vi "COMMAND_ChangeVelocity.vi"(8 "error in (no error)":errorcluster, 10 "velocity":dbl[unit], 11 "StageDL090602SutterMP285 in":refnum<class "StageMMS2015ASI.lvclass">) -> (0 "error out":errorcluster, 3 "StageDL090602SutterMP285 out":refnum<class "StageMMS2015ASI.lvclass">)   [LabVIEW 2010, in "StageMMS2015ASI.lvclass"]
uses:
  StageMMS2015ASI.lvclass
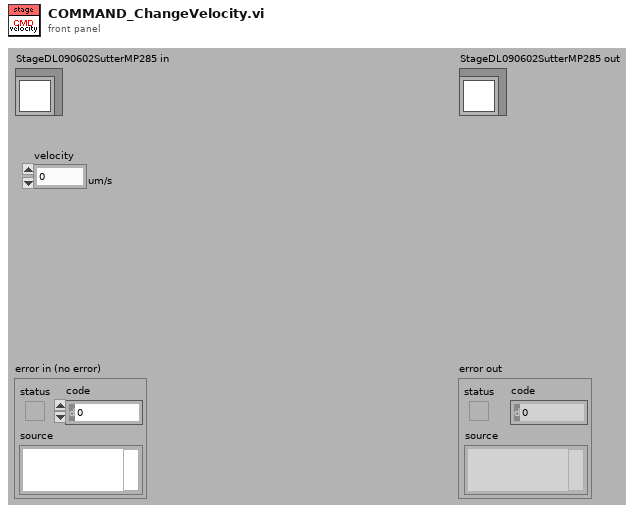
[diagram p1: front panel]
types:
  T1 = typedef "StageMMS2015ASI.lvclass/status_cluster.ctl" = cluster{"STEP_DIV":i32, "STEP_MUL":i32, "XSPEED":i32, "VERSION":i32}
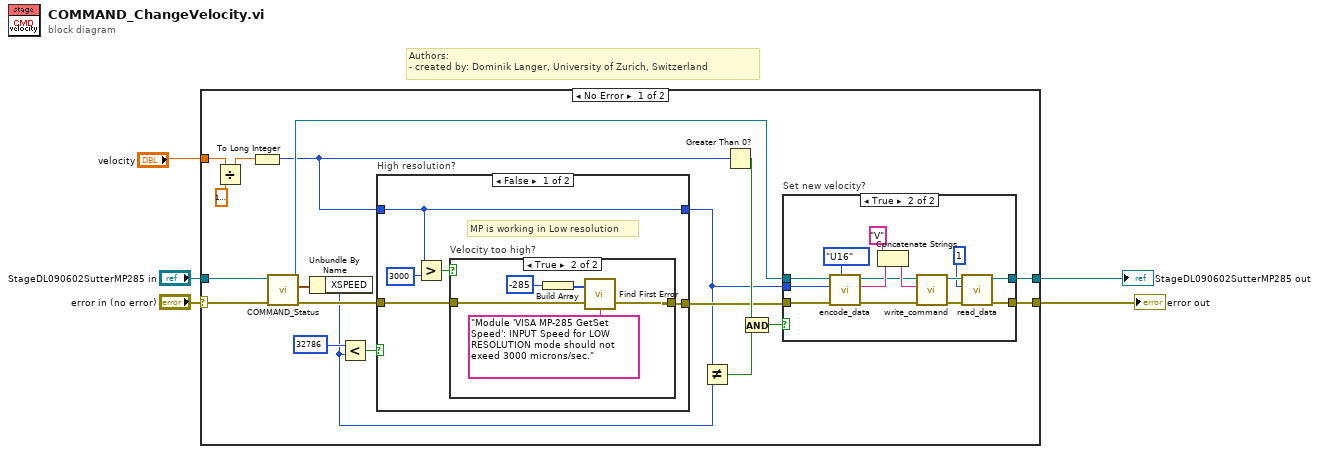
[diagram p0: block diagram]
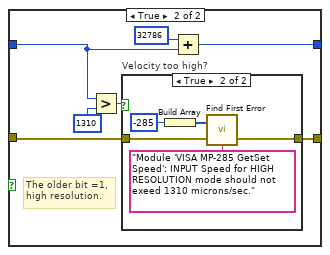
[diagram p4: hidden frame]
diagram:
  # "Authors: \n- created by: Dominik Langer, University of Zurich, Switzerland"
  n1 = case shown="No Error" "error in (no error)" {
    selector: "error in (no error)" -> [w24 w66]
    tunnel: [w22 w66] -> w4
    tunnel: [w21 w65] -> w2
    tunnel: "StageDL090602SutterMP285 in" -> [w23 w65]
    tunnel: "velocity" -> [w9 _]
    frame No Error {
      n2 = Divide(x=w9, y=dbl[unit] 1e-06) -> (x/y=w8:dbl)
      n3 = To Long Integer(number=w8) -> (32bit integer=w7:i32)
      n4 = call-dynamic "COMMAND_Status.vi"("error in (no error)"=w24, "StageDL090602SutterMP285 in"=w23) -> ("error out"=w14:errorcluster, "status"=w20:T1, "StageDL090602SutterMP285 out"=w11:refnum<class "StageMMS2015ASI.lvclass">)  [unwired: 7 in]
      n5 = Unbundle By Name(w20) -> ("XSPEED"=w12:i32)
      n6 = Less?(x=32786, y=w12) -> (x < y?=w19:bool)
      n7 = case "High resolution?" shown="False" w19 {
        tunnel: [w41 w53] -> w6
        tunnel: w7 -> [w41 w52]
        tunnel: w14 -> [w43 w55]
        tunnel: [w42 w54] -> w13
        frame False {
          # "MP is working in Low resolution"
          n8 = Greater?(x=w41, y=3000) -> (0:w44:bool)
          n9 = case "Velocity too high?" shown="True" w44 {
            tunnel: w43 -> [w46 w51]
            tunnel: [w46 w50] -> w42
            frame False {
              # "An INPUT is\nin range."
            }
            frame True {
              n10 = Build Array(-285) -> (w49:i32[])
              n11 = call <vilib>:"Find First Error.vi"("error in (no error)"=w51, "source messages"="Module 'VISA MP-285 GetSet Speed': INPUT Speed for LOW RESOLUTION mode should not exeed 3000 microns/sec.", "error codes"=w49) -> ("error out"=w50:errorcluster)  [unwired: 1 in, 1 out]
            }
          }
        }
        frame True {
          # "The older bit =1, \nhigh resolution."
          n12 = Greater?(x=w52, y=1310) -> (0:w57:bool)
          n13 = case "Velocity too high?" shown="True" w57 {
            tunnel: w55 -> [w59 w63]
            tunnel: [w59 w64] -> w54
            frame False {
              # "Input correct, \nWe can write."
            }
            frame True {
              n14 = Build Array(-285) -> (w61:i32[])
              n15 = call <vilib>:"Find First Error.vi"("error in (no error)"=w63, "source messages"="Module 'VISA MP-285 GetSet Speed': INPUT Speed for HIGH RESOLUTION mode should not exeed 1310 microns/sec.", "error codes"=w61) -> ("error out"=w64:errorcluster)  [unwired: 1 in, 1 out]
            }
          }
          n16 = Add(x=32786, y=w52) -> (x+y=w53:i32)
        }
      }
      n17 = Not Equal?(x=w6, y=w12) -> (x != y?=w17:bool)
      n18 = Greater Than 0?(x=w7) -> (x > 0?=w16:bool)
      n19 = And(x=w16, y=w17) -> (x .and. y?=w15:bool)
      n20 = case "Set new velocity?" shown="True" w15 {
        tunnel: w13 -> [w25 w40]
        tunnel: [w25 w29] -> w22
        tunnel: w11 -> [w26 w39]
        tunnel: [w26 w28] -> w21
        tunnel: w6 -> [_ w32]
        frame False {
        }
        frame True {
          n21 = call-dynamic "encode_data.vi"("data type"=enum16{"U16", "I32"}."U16", "error in (no error)"=w40, "data I32"=w32, "DL090602SutterMP285Stage in"=w39) -> ("error out"=w33:errorcluster, "encoded data"=w37:string, "DL090602SutterMP285Stage out"=w34:refnum<class "StageMMS2015ASI.lvclass">)  [unwired: 5 out]
          n22 = Concatenate Strings("V" ("string"), w37) -> (w35:string)
          n23 = call-dynamic "write_command.vi"("error in (no error)"=w33, "command (without terminating \"\\n\")"=w35, "DL090602SutterMP285Stage in"=w34) -> ("error out"=w31:errorcluster, "DL090602SutterMP285Stage out"=w30:refnum<class "StageMMS2015ASI.lvclass">)  [unwired: 7 in]
          n24 = call-dynamic "read_data.vi"("error in (no error)"=w31, "bytes to read"=u32 1, "DL090602SutterMP285Stage in"=w30) -> ("error out"=w29:errorcluster, "DL090602SutterMP285Stage out"=w28:refnum<class "StageMMS2015ASI.lvclass">)  [unwired: 6 in, 1 out]
        }
      }
    }
    frame Error {
    }
  }
  "error out" <- w4
  "StageDL090602SutterMP285 out" <- w2
